vi "Destroy.vi"(8 "Error In":errorcluster, 11 "KnownHosts":refnum<class "KnownHosts.lvclass">) -> (0 "Error Out":errorcluster, 3 "Session":refnum<class "Session.lvclass">)   [LabVIEW 2017, in "LabSSH2.lvlib" / "KnownHosts.lvclass"]
uses:
  KnownHosts.lvclass
  Session/Session.lvclass
  KnownHosts.lvclass/KnownHosts.ctl
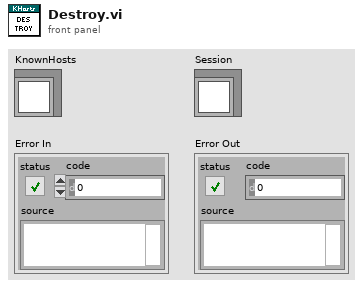
[diagram p1: front panel]
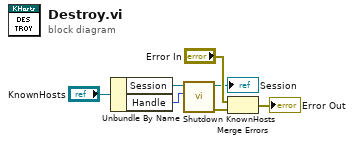
[diagram p0: block diagram]
diagram:
  n1 = Unbundle By Name("KnownHosts") -> ("Session"=w3:refnum<class "Session.lvclass">, "Handle"=w4:u64)
  n2 = call "Shutdown KnownHosts.vi"("Handle"=w4, "Session In"=w3) -> ("Error Out"=w2:errorcluster, "Session Out"=→"Session":refnum<class "Session.lvclass">)  [unwired: 8 in]
  n3 = Merge Errors("Error In", w2) -> (→"Error Out":errorcluster)
